vi "Exercise 4-1.vi"(8 "Min Temp":dbl, 9 "Max Temp":dbl, 10 "Current Temp":dbl) -> (1 "Warning?":bool, 2 "Warning Text":string)   [LabVIEW 2014]
panel:
  out "error out":errorcluster
  in  "error in (no error)":errorcluster
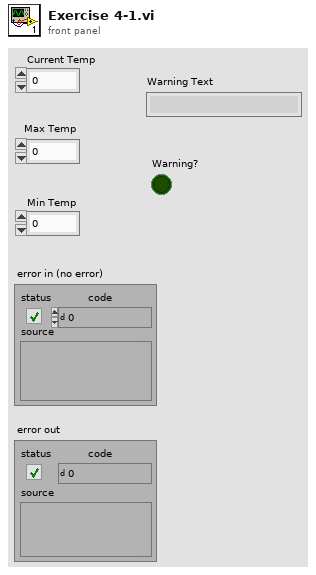
[diagram p1: front panel]
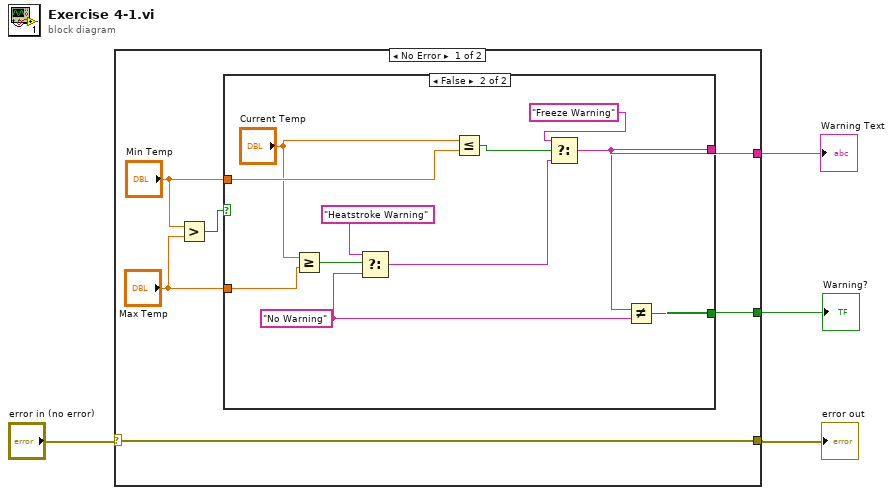
[diagram p0: block diagram]
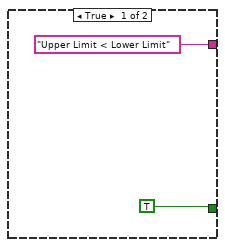
[diagram p2: hidden frame]
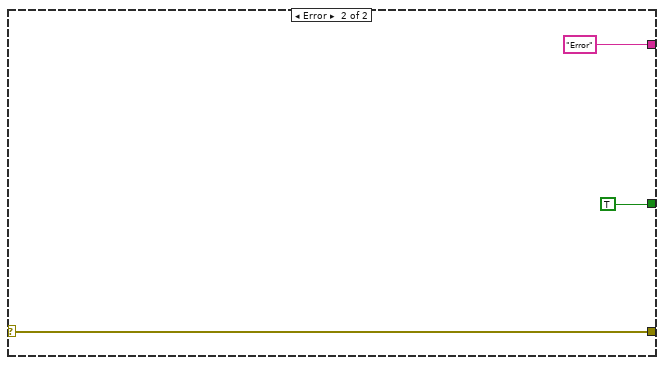
[diagram p3: hidden frame]
diagram:
  n1 = case shown="No Error" "error in (no error)" {
    selector: "error in (no error)" -> [w5 w26]
    tunnel: [w10 TRUE] -> w4
    tunnel: [w9 "Error"] -> w3
    tunnel: [w5 w26] -> w1
    frame No Error {
      n2 = Greater?(x="Min Temp", y="Max Temp") -> (0:w8:bool)
      n3 = case shown="False" w8 {
        tunnel: [TRUE w21] -> w10
        tunnel: ["Upper Limit < Lower Limit" w20] -> w9
        tunnel: "Max Temp" -> [_ w18]
        tunnel: "Min Temp" -> [_ w16]
        frame True {
        }
        frame False {
          w13 = "No Warning" ("String")
          n4 = Greater Or Equal?(x="Current Temp", y=w18) -> (x >= y?=w14:bool)
          n5 = Select(t="Heatstroke Warning" ("String"), s=w14, f=w13) -> (s? t:f=w19:string)
          n6 = Less Or Equal?(x="Current Temp", y=w16) -> (x <= y?=w23:bool)
          n7 = Select(t="Freeze Warning" ("String"), s=w23, f=w19) -> (s? t:f=w20:string)
          n8 = Not Equal?(x=w20, y=w13) -> (x != y?=w21:bool)
        }
      }
    }
    frame Error {
    }
  }
  "Warning Text" <- w3
  "Warning?" <- w4
  "error out" <- w1
